vi "Configure.vi"(8 "error in (no error)":errorcluster, 10 "SPI User Configuration":T1={"Frequency [Hz]"=1000000.0, "Clock Phase"=enum."Leading", "Clock Polarity"=enum."Low", "Data Direction"=enum."Most significant bit first", "Frame Length"=8} {"Frame Length" min=1 max=16}, 11 "SPI Ref In":T6={"myRIO Reference"={"myRIO Model"=enum."Unknown", "myRIO Hardware Reference"={"Generic FPGA Reference"=refnum, "Allow multiple opens"=FALSE}}, "SPI Channels Enum"=enum."Not Connected", "SPI Configuration"={"Frequency [Hz]"=0.0, "Clock Phase"=enum."Leading", "Clock Polarity"=enum."Low", "Data Direction"=enum."Most significant bit first", "Frame Length"=8}} {"SPI Configuration"."Frame Length" min=1 max=16}) -> (0 "error out":errorcluster, 3 "SPI Ref Out":T6={"myRIO Reference"={"myRIO Model"=enum."Unknown", "myRIO Hardware Reference"={"Generic FPGA Reference"=refnum, "Allow multiple opens"=FALSE}}, "SPI Channels Enum"=enum."Not Connected", "SPI Configuration"={"Frequency [Hz]"=0.0, "Clock Phase"=enum."Leading", "Clock Polarity"=enum."Low", "Data Direction"=enum."Most significant bit first", "Frame Length"=8}} {"SPI Configuration"."Frame Length" min=1 max=16})   [LabVIEW 2021, in "SPI.lvlib"]
doc: "Configures a serial peripheral interface (SPI) channel based on the input SPI reference and the user configurations that you specify."
uses:
  <vilib>/myRIO/Instrument Drivers/Onboard IO/SPI/SPI.lvlib
  <vilib>/myRIO/Instrument Drivers/Onboard IO/SPI/typedefs/SPI Reference.ctl
  <vilib>/myRIO/Common/Instrument Driver Framework/Utilities/typedefs/myRIO Generic Hardware Reference.ctl
  <vilib>/myRIO/Common/Instrument Driver Framework/Utilities/typedefs/Hardware Version Enum.ctl
  <vilib>/myRIO/Common/Instrument Driver Framework/Utilities/typedefs/myRIO v1.0 Reference.ctl
  <vilib>/myRIO/Common/Instrument Driver Framework/Utilities/typedefs/Generic FPGA Reference.ctl
  <vilib>/myRIO/Common/Instrument Driver Framework/myRIO v1.0/SPI/typedefs/SPI Channels Enum.ctl
  <vilib>/myRIO/Instrument Drivers/Onboard IO/SPI/typedefs/SPI Configuration.ctl
  <vilib>/myRIO/Common/Instrument Driver Framework/myRIO v1.0/SPI/typedefs/SPI Clock Phase.ctl
  <vilib>/myRIO/Common/Instrument Driver Framework/myRIO v1.0/SPI/typedefs/SPI Clock Polarity.ctl
  <vilib>/myRIO/Common/Instrument Driver Framework/myRIO v1.0/SPI/typedefs/SPI Data Direction.ctl
  <vilib>/myRIO/Common/Instrument Driver Framework/myRIO v1.0/SPI/typedefs/SPI Frame Length.ctl
  <vilib>/myRIO/Instrument Drivers/Onboard IO/SPI/typedefs/SPI User Configuration.ctl
  <vilib>/myRIO/Common/Instrument Driver Framework/myRIO v1.0/SPI/typedefs/SPI Configuration v1.0.ctl
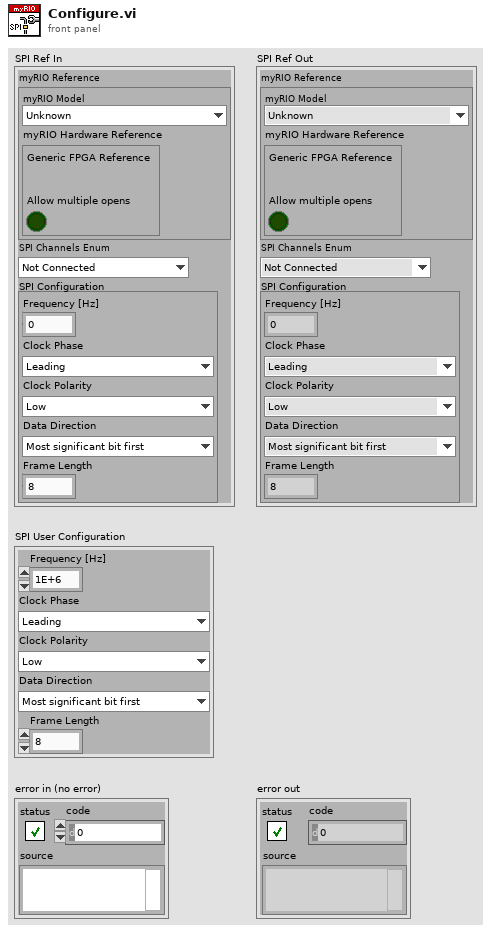
[diagram p1: front panel]
types:
  T1 = typedef "SPI.lvlib/SPI User Configuration.ctl" = cluster{"Frequency [Hz]":dbl, "Clock Phase":T2, "Clock Polarity":T3, "Data Direction":T4, "Frame Length":T5}
  T2 = typedef "SPI Clock Phase.ctl" = enum8{"Leading", "Trailing"}
  T3 = typedef "SPI Clock Polarity.ctl" = enum8{"Low", "High"}
  T4 = typedef "SPI Data Direction.ctl" = enum8{"Most significant bit first", "Least significant bit first"}
  T5 = typedef "SPI Frame Length.ctl" = u8
  T6 = typedef "SPI.lvlib/SPI Reference.ctl" = cluster{"myRIO Reference":T7, "SPI Channels Enum":T11, "SPI Configuration":T12}
  T7 = typedef "myRIO Generic Hardware Reference.ctl" = cluster{"myRIO Model":T8, "myRIO Hardware Reference":T9}
  T8 = typedef "Hardware Version Enum.ctl" = enum16{"Unknown", "myRIO-1900", "myRIO-1950", "roboRIO", "NI ELVIS RIO CM", "ELVIS III"}
  T9 = typedef "myRIO v1.0 Reference.ctl" = cluster{"Generic FPGA Reference":T10, "Allow multiple opens":bool}
  T10 = typedef "Generic FPGA Reference.ctl" = refnum<k20>
  T11 = typedef "SPI Channels Enum.ctl" = enum16{"Not Connected", "A/SPI", "B/SPI", "SPI/SPI"}
  T12 = typedef "SPI.lvlib/SPI Configuration.ctl" = cluster{"Frequency [Hz]":dbl, "Clock Phase":T2, "Clock Polarity":T3, "Data Direction":T4, "Frame Length":T5}
  T13 = typedef "SPI Configuration v1.0.ctl" = cluster{"Frequency (Hz)":dbl, "SPI Clock Phase":T2, "SPI Clock Polarity":T3, "SPI Data Direction":T4, "Frame Length":T5}
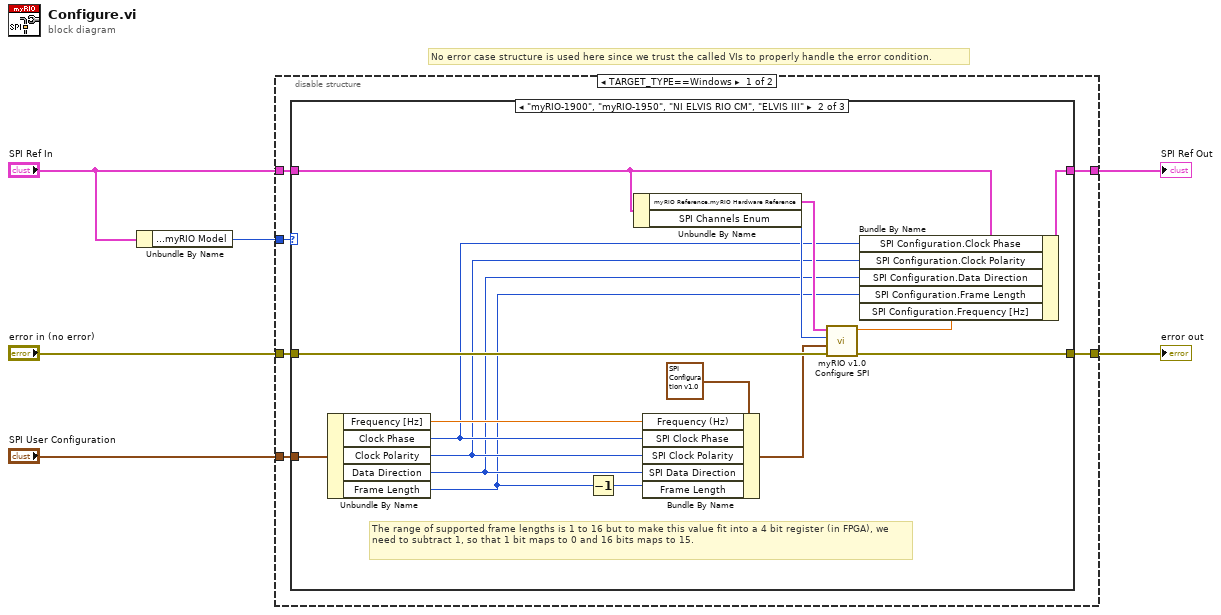
[diagram p0: block diagram]
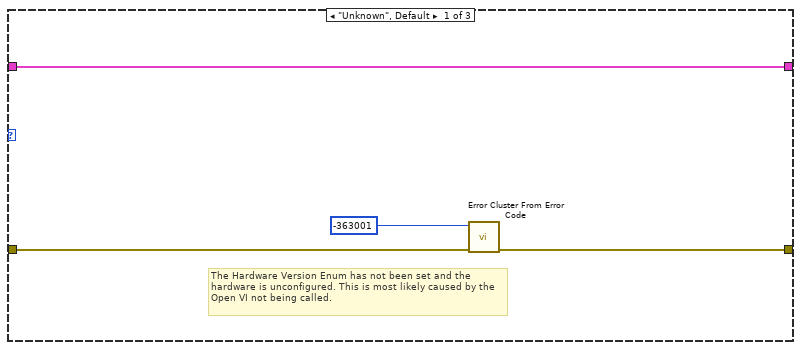
[diagram p2: hidden frame]
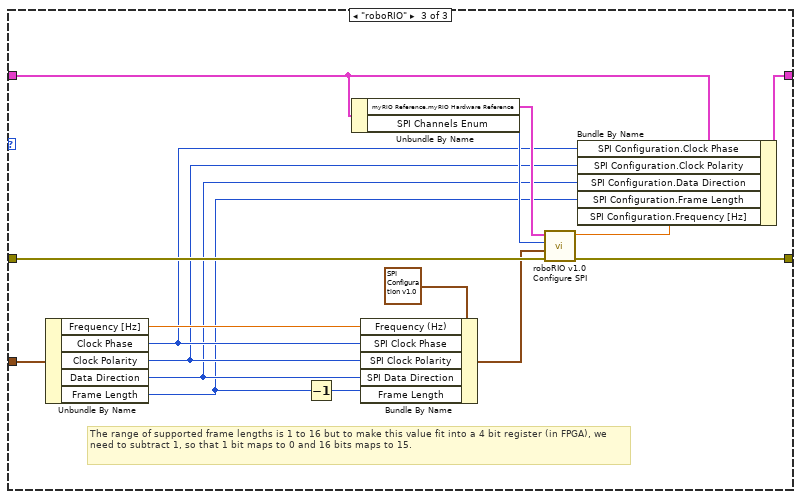
[diagram p3: hidden frame]
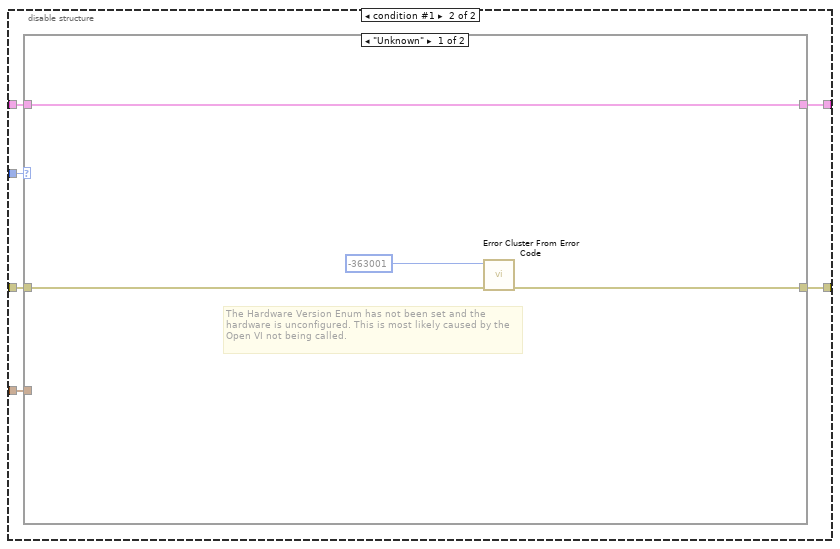
[diagram p4: hidden frame]
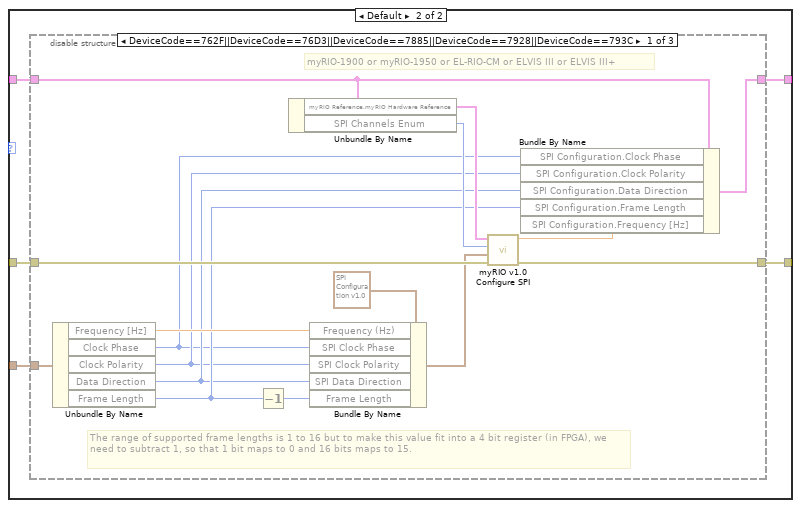
[diagram p5: hidden frame]
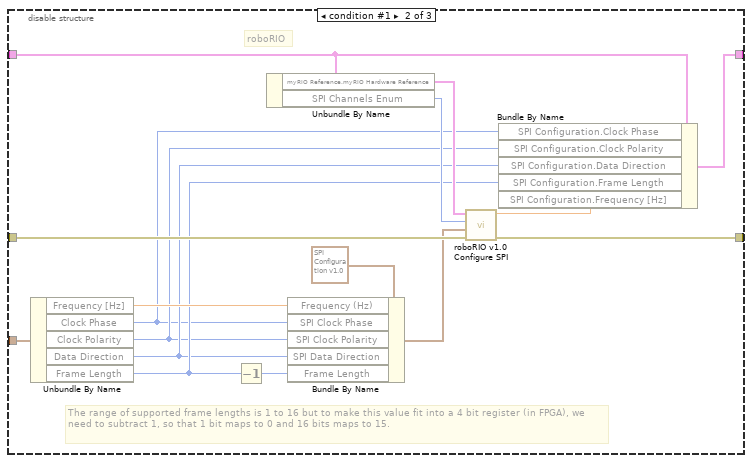
[diagram p6: hidden frame]
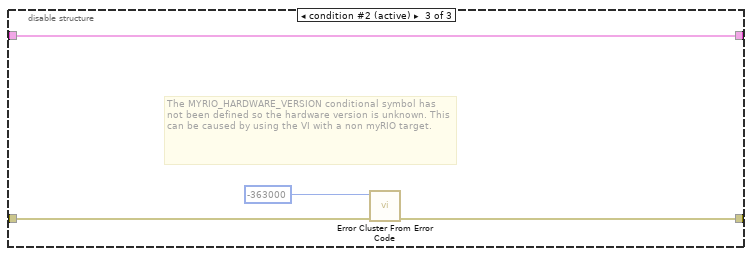
[diagram p7: hidden frame]
diagram:
  # "No error case structure is used here since we trust the called VIs to properly handle the error condition."
  n1 = Unbundle By Name("SPI Ref In") -> ("myRIO Reference.myRIO Model"=w1:T8)
  n2 = disable-structure shown="TARGET_TYPE==Windows" {
    disable-tunnel: [w12 w54] -> w6
    disable-tunnel: [w11 w53] -> w5
    disable-tunnel: "SPI User Configuration" -> [w10 w52]
    disable-tunnel: "SPI Ref In" -> [w9 w51]
    disable-tunnel: "error in (no error)" -> [w8 w50]
    disable-tunnel: w1 -> [w7 w49]
    frame condition #0 (active) {
      n3 = case shown="\"myRIO-1900\", \"myRIO-1950\", \"NI ELVIS RIO CM\", \"ELVIS III\"" w7 {
        tunnel: [w15 w32 w48] -> w12
        tunnel: [w14 w18 w34] -> w11
        tunnel: w9 -> [w14 w19 w35]
        tunnel: w8 -> [w13 w30 w46]
        tunnel: w10 -> [_ w25 w41]
        frame "Unknown", Default {
          # "The Hardware Version Enum has not been set and the hardware is unconfigured. This is most likely caused by the Open VI not being called."
          n4 = call <vilib>:"Error Cluster From Error Code.vi"("error in (no error)"=w13, "error code (0)"=-363001) -> ("error out"=w15:errorcluster)  [unwired: 7 in]
        }
        frame "myRIO-1900", "myRIO-1950", "NI ELVIS RIO CM", "ELVIS III" {
          # "The range of supported frame lengths is 1 to 16 but to make this value fit into a 4 bit register (in FPGA), we need to subtract 1, so that 1 bit maps to 0 and 16 bits maps to 15."
          n5 = Unbundle By Name(w25) -> ("Frequency [Hz]"=w24:dbl, "Clock Phase"=w23:T2, "Clock Polarity"=w22:T3, "Data Direction"=w21:T4, "Frame Length"=w20:T5)
          n6 = Decrement(x=w20) -> (x-1=w29:T5)
          n7 = Unbundle By Name(w19) -> ("myRIO Reference.myRIO Hardware Reference"=w27:T9, "SPI Channels Enum"=w28:T11)
          n8 = Bundle By Name(cluster=T13 {"Frequency (Hz)"=0.0, "SPI Clock Phase"=enum."Leading", "SPI Clock Polarity"=enum."Low", "SPI Data Direction"=enum."Most significant bit first", "Frame Length"=0} ("SPI Configuration"), "Frequency (Hz)"=w24, "SPI Clock Phase"=w23, "SPI Clock Polarity"=w22, "SPI Data Direction"=w21, "Frame Length"=w29) -> (w26:T13)
          n9 = call <vilib>:"myRIO v1.0 Configure SPI.vi"("error in (no error)"=w30, "SPI Configuration v1.0"=w26, "SPI Channel"=w28, "myRIO Ref In"=w27) -> ("error out"=w32:errorcluster, "Actual Frequency (Hz)"=w17:dbl)  [unwired: 6 in]
          n10 = Bundle By Name(cluster=w19, "SPI Configuration.Clock Phase"=w23, "SPI Configuration.Clock Polarity"=w22, "SPI Configuration.Data Direction"=w21, "SPI Configuration.Frame Length"=w20, "SPI Configuration.Frequency [Hz]"=w17) -> (w18:T6)
        }
        frame "roboRIO" {
          # "The range of supported frame lengths is 1 to 16 but to make this value fit into a 4 bit register (in FPGA), we need to subtract 1, so that 1 bit maps to 0 and 16 bits maps to 15."
          n11 = Unbundle By Name(w41) -> ("Frequency [Hz]"=w40:dbl, "Clock Phase"=w39:T2, "Clock Polarity"=w38:T3, "Data Direction"=w37:T4, "Frame Length"=w36:T5)
          n12 = Decrement(x=w36) -> (x-1=w45:T5)
          n13 = Unbundle By Name(w35) -> ("myRIO Reference.myRIO Hardware Reference"=w43:T9, "SPI Channels Enum"=w44:T11)
          n14 = Bundle By Name(cluster=T13 {"Frequency (Hz)"=0.0, "SPI Clock Phase"=enum."Leading", "SPI Clock Polarity"=enum."Low", "SPI Data Direction"=enum."Most significant bit first", "Frame Length"=0} ("SPI Configuration"), "Frequency (Hz)"=w40, "SPI Clock Phase"=w39, "SPI Clock Polarity"=w38, "SPI Data Direction"=w37, "Frame Length"=w45) -> (w42:T13)
          n15 = call <vilib>:"roboRIO v1.0 Configure SPI.vi"("error in (no error)"=w46, "SPI Configuration v1.0"=w42, "SPI Channel"=w44, "myRIO Ref In"=w43) -> ("error out"=w48:errorcluster, "Actual Frequency (Hz)"=w33:dbl)  [unwired: 6 in]
          n16 = Bundle By Name(cluster=w35, "SPI Configuration.Clock Phase"=w39, "SPI Configuration.Clock Polarity"=w38, "SPI Configuration.Data Direction"=w37, "SPI Configuration.Frame Length"=w36, "SPI Configuration.Frequency [Hz]"=w33) -> (w34:T6)
        }
      }
    }
    frame condition #1 {
      n17 = case shown="\"Unknown\"" w49 {
        tunnel: [w57 w63] -> w54
        tunnel: [w56 w62] -> w53
        tunnel: w51 -> [w56 w60]
        tunnel: w50 -> [w55 w61]
        tunnel: w52 -> [_ w59]
        frame "Unknown" {
          # "The Hardware Version Enum has not been set and the hardware is unconfigured. This is most likely caused by the Open VI not being called."
          n18 = call <vilib>:"Error Cluster From Error Code.vi"("error in (no error)"=w55, "error code (0)"=-363001) -> ("error out"=w57:errorcluster)  [unwired: 7 in]
        }
        frame Default {
          n19 = disable-structure shown="DeviceCode==762F||DeviceCode==76D3||DeviceCode==7885||DeviceCode==7928||DeviceCode==793C" {
            disable-tunnel: [w79 w95 w96] -> w63
            disable-tunnel: [w65 w81 w99] -> w62
            disable-tunnel: w61 -> [w77 w93 w97]
            disable-tunnel: w60 -> [w66 w82 w99]
            disable-tunnel: w59 -> [w72 w88 _]
            frame condition #0 {
              # "myRIO-1900 or myRIO-1950 or EL-RIO-CM or ELVIS III or ELVIS III+"
              # "The range of supported frame lengths is 1 to 16 but to make this value fit into a 4 bit register (in FPGA), we need to subtract 1, so that 1 bit maps to 0 and 16 bits maps to 15."
              n20 = Unbundle By Name(w72) -> ("Frequency [Hz]"=w71:dbl, "Clock Phase"=w67:T2, "Clock Polarity"=w68:T3, "Data Direction"=w69:T4, "Frame Length"=w70:T5)
              n21 = Decrement(x=w70) -> (x-1=w76:T5)
              n22 = Unbundle By Name(w66) -> ("myRIO Reference.myRIO Hardware Reference"=w74:T9, "SPI Channels Enum"=w75:T11)
              n23 = Bundle By Name(cluster=T13 {"Frequency (Hz)"=0.0, "SPI Clock Phase"=enum."Leading", "SPI Clock Polarity"=enum."Low", "SPI Data Direction"=enum."Most significant bit first", "Frame Length"=0} ("SPI Configuration"), "Frequency (Hz)"=w71, "SPI Clock Phase"=w67, "SPI Clock Polarity"=w68, "SPI Data Direction"=w69, "Frame Length"=w76) -> (w73:T13)
              n24 = call <vilib>:"myRIO v1.0 Configure SPI.vi"("error in (no error)"=w77, "SPI Configuration v1.0"=w73, "SPI Channel"=w75, "myRIO Ref In"=w74) -> ("error out"=w79:errorcluster, "Actual Frequency (Hz)"=w64:dbl)  [unwired: 6 in]
              n25 = Bundle By Name(cluster=w66, "SPI Configuration.Clock Phase"=w67, "SPI Configuration.Clock Polarity"=w68, "SPI Configuration.Data Direction"=w69, "SPI Configuration.Frame Length"=w70, "SPI Configuration.Frequency [Hz]"=w64) -> (w65:T6)
            }
            frame condition #1 {
              # "roboRIO"
              # "The range of supported frame lengths is 1 to 16 but to make this value fit into a 4 bit register (in FPGA), we need to subtract 1, so that 1 bit maps to 0 and 16 bits maps to 15."
              n26 = Unbundle By Name(w88) -> ("Frequency [Hz]"=w87:dbl, "Clock Phase"=w83:T2, "Clock Polarity"=w84:T3, "Data Direction"=w85:T4, "Frame Length"=w86:T5)
              n27 = Decrement(x=w86) -> (x-1=w92:T5)
              n28 = Unbundle By Name(w82) -> ("myRIO Reference.myRIO Hardware Reference"=w90:T9, "SPI Channels Enum"=w91:T11)
              n29 = Bundle By Name(cluster=T13 {"Frequency (Hz)"=0.0, "SPI Clock Phase"=enum."Leading", "SPI Clock Polarity"=enum."Low", "SPI Data Direction"=enum."Most significant bit first", "Frame Length"=0} ("SPI Configuration"), "Frequency (Hz)"=w87, "SPI Clock Phase"=w83, "SPI Clock Polarity"=w84, "SPI Data Direction"=w85, "Frame Length"=w92) -> (w89:T13)
              n30 = call <vilib>:"roboRIO v1.0 Configure SPI.vi"("error in (no error)"=w93, "SPI Configuration v1.0"=w89, "SPI Channel"=w91, "myRIO Ref In"=w90) -> ("error out"=w95:errorcluster, "Actual Frequency (Hz)"=w80:dbl)  [unwired: 6 in]
              n31 = Bundle By Name(cluster=w82, "SPI Configuration.Clock Phase"=w83, "SPI Configuration.Clock Polarity"=w84, "SPI Configuration.Data Direction"=w85, "SPI Configuration.Frame Length"=w86, "SPI Configuration.Frequency [Hz]"=w80) -> (w81:T6)
            }
            frame condition #2 (active) {
              # "The MYRIO_HARDWARE_VERSION conditional symbol has not been defined so the hardware version is unknown. This can be caused by using the VI with a non myRIO target."
              n32 = call <vilib>:"Error Cluster From Error Code.vi"("error in (no error)"=w97, "error code (0)"=-363000) -> ("error out"=w96:errorcluster)  [unwired: 7 in]
            }
          }
        }
      }
    }
  }
  "SPI Ref Out" <- w5
  "error out" <- w6
